vi "wait_nre.vi"(0 "wait_ms":u32=1000) -> ()   [LabVIEW 2015, in "lv_mutex_shared_1.lvlib"]
uses:
  lv_mutex_shared_1.lvlib
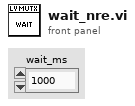
[diagram p1: front panel]
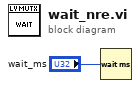
[diagram p0: block diagram]
diagram:
  n1 = Wait (ms)(milliseconds to wait="wait_ms") -> ()  [unwired: 1 out]
